vi "NXTLineLeader-DC.vi"(3 "Select your \nInput Port":T2 items=["Port 1", "Port 2", "Port 3", "Port 4"], 5 "NXT":T1={"error"={"status"=FALSE, "code"=0, "source"=""}, "address"="", "NXT #"=-1, "Show Error"=TRUE}) -> (17 "Boolean array":bool[](array[boolean]), 19 "NXT dup":T1={"error"={"status"=FALSE, "code"=0, "source"=""}, "address"="", "NXT #"=-1, "Show Error"=TRUE}, 20 "Sensor 1 Reading":u8, 21 "Sensor 2 Reading":u8, 22 "Sensor 3 Reading":u8, 23 "Sensor 4 Reading":u8, 24 "Sensor 5 Reading":u8, 25 "Sensor 6 Reading":u8, 26 "Sensor 7 Reading":u8, 27 "Sensor 8 Reading":u8)   [LabVIEW 2009]
uses:
  <vilib>/NXT/Block Support/NXT_InputPort.ctl
  <vilib>/NXT/Subs/LVHSConnector.ctl
  <vilib>/NXT/Block Support/HWPage.SensorType.ctl
  <vilib>/NXT/Block Support/HWPage.SensorMode.ctl
panel:
  # "mindsensors.com\nCopyright (c) 2009 by mindsensors.com\nEmail: info (<at>) mindsensors (<dot>) com\n\nThis program is free software. You can redistribute it and/or modify\nit under the terms of the GNU General Public License as published by\nthe Free Software Foundation; version 3 of the License.\nRead the license at: http://www.gnu.org/licenses/gpl.txt"
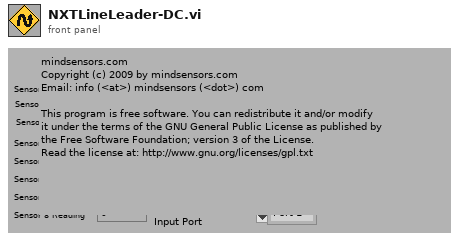
[diagram p1: front panel]
types:
  T1 = typedef "LVHSConnector.ctl" = cluster{"error":errorcluster, "address":string, "NXT #":i32, "Show Error":bool}
  T2 = typedef "NXT_InputPort.ctl" = u8
  T3 = typedef "HWPage.SensorMode.ctl" = u8
  T4 = typedef "HWPage.SensorType.ctl" = u8
  T5 = typedef "nxt.ctl" = cluster{"nxtHandle":u32, "fileHandle":u32, "fileIterHandle":u32, "moduleHandle":u32, "modIterHandle":u32, "nxtIterHandle":u32}
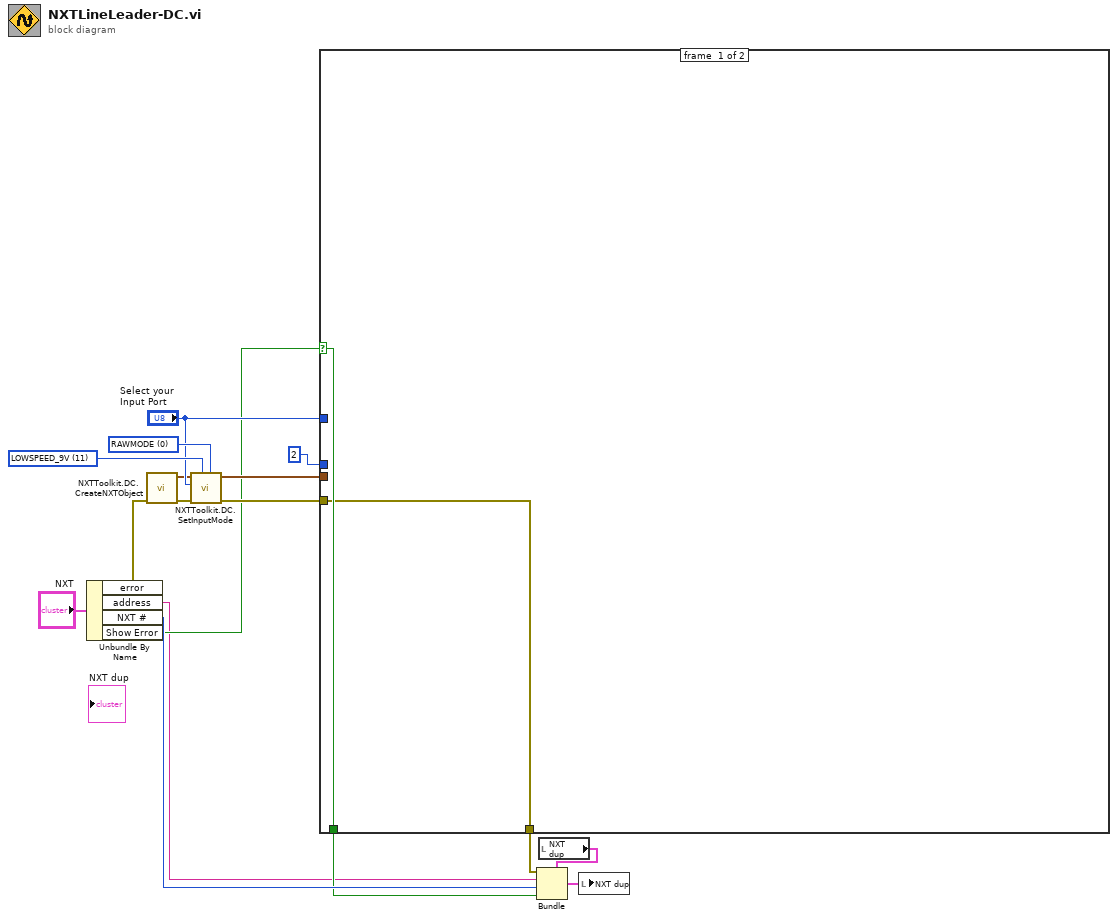
[diagram p0: block diagram]
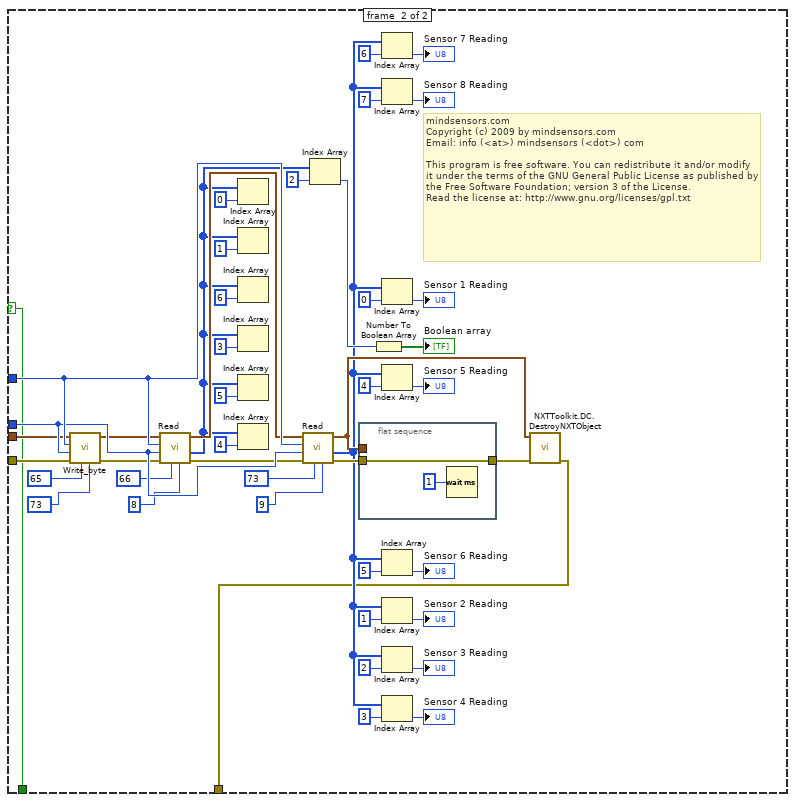
[diagram p2: hidden frame]
diagram:
  w15 = T3 0 items=["RAWMODE"=0, "BOOLEANMODE"=32, "TRANSITIONCNTMODE"=64, "PERIODCOUNTERMODE"=96, "PCTFULLSCALEMODE"=128, "CELSIUSMODE"=160, "FAHRENHEITMODE"=192, "ANGLESTEPMODE"=224] ("Sensor Mode (RAWMODE)")
  w16 = T4 11 items=["NO_SENSOR", "SWITCH", "TEMPERATURE", "REFLECTION", "ANGLE", "LIGHT_ACTIVE", "LIGHT_INACTIVE", "SOUND_DB", "SOUND_DBA", "CUSTOM", "LOWSPEED", "LOWSPEED_9V", "HIGHSPEED"] ("Sensor Type (NO_SENSOR)")
  n1 = Unbundle By Name("NXT") -> ("error"=w3:errorcluster, "address"=w4:string, "NXT #"=w7:i32, "Show Error"=w5:bool)
  n2 = call <vilib>:"NXTToolkit.DC.CreateNXTObject.vi"("error in (no error)"=w3) -> ("error out"=w17:errorcluster, "NXTObject"=w11:T5)  [unwired: 8 in, 1 out]
  n3 = call <vilib>:"NXTToolkit.DC.SetInputMode.vi"("Sensor Mode (RAWMODE)"=w15, "Sensor Type (NO_SENSOR)"=w16, "error in (no error)"=w17, "Input Port (Port 1)"="Select your \nInput Port", "NXTObject"=w11) -> ("error out"=w12:errorcluster, "NXTObject dup"=w13:T5)  [unwired: 4 in, 1 out]
  n4 = case shown="True" w5 {
    selector: w5 -> [w19 w21]
    tunnel: "Select your \nInput Port" -> [_ w63]
    tunnel: 2 -> [_ w62]
    tunnel: w13 -> [_ w59]
    tunnel: w12 -> [w18 w58]
    tunnel: [w19 w21] -> w6
    tunnel: [w18 w20] -> w2
    frame #0 {
    }
    frame #1 {
      # "mindsensors.com\nCopyright (c) 2009 by mindsensors.com\nEmail: info (<at>) mindsensors (<dot>) com\n\nThis program is free software. You can redistribute it and/or modify\nit under the terms of the GNU General Public License as published by\nthe Free Software Foundation; version 3 of the License.\nRead the license at: http://www.gnu.org/licenses/gpl.txt"
      n5 = call "Write_byte.vi"("Data byte"=73, "Reg Address"=u8 65, "error in (no error)"=w58, "Device Address"=w62, "Input Port in"=w63, "NXTObject"=w59) -> ("error out"=w60:errorcluster, "NXTObject dup"=w61:T5)  [unwired: 1 in, 3 out]
      n6 = call "Read.vi"("bytes to read"=u8 8, "Reg Address"=u8 66, "error in (no error)"=w60, "Device Address"=w62, "Input Port in"=w63, "NXTObject"=w61) -> ("error out"=w26:errorcluster, "data Buffer"=w24:u8[], "NXTObject dup"=w27:T5)  [unwired: 3 out]
      n7 = Index Array(array=w24, index=0) -> ()  [unwired: 1 out]
      n8 = Index Array(array=w24, index=1) -> ()  [unwired: 1 out]
      n9 = Index Array(array=w24, index=6) -> ()  [unwired: 1 out]
      n10 = Index Array(array=w24, index=3) -> ()  [unwired: 1 out]
      n11 = Index Array(array=w24, index=5) -> ()  [unwired: 1 out]
      n12 = Index Array(array=w24, index=4) -> ()  [unwired: 1 out]
      n13 = call "Read.vi"("bytes to read"=u8 9, "Reg Address"=u8 73, "error in (no error)"=w26, "Device Address"=w62, "Input Port in"=w63, "NXTObject"=w27) -> ("error out"=w52:errorcluster, "data Buffer"=w23:u8[], "NXTObject dup"=w57:T5)  [unwired: 3 out]
      n14 = Index Array(array=w24, index=2) -> (element=w36:u8)
      n15 = flat-sequence {
        tunnel: [w66] -> w22
        tunnel: w52 -> [w66]
        tunnel: w57 -> [_]
        frame #0 {
          n16 = Wait (ms)(milliseconds to wait=u32 1) -> ()  [unwired: 1 out]
        }
      }
      n17 = Number To Boolean Array(number=w36) -> (Boolean array=→"Boolean array":bool[])
      n18 = Index Array(array=w23, index=6) -> (element=→"Sensor 7 Reading":u8)
      n19 = Index Array(array=w23, index=7) -> (element=→"Sensor 8 Reading":u8)
      n20 = Index Array(array=w23, index=0) -> (element=→"Sensor 1 Reading":u8)
      n21 = Index Array(array=w23, index=4) -> (element=→"Sensor 5 Reading":u8)
      n22 = Index Array(array=w23, index=5) -> (element=→"Sensor 6 Reading":u8)
      n23 = Index Array(array=w23, index=1) -> (element=→"Sensor 2 Reading":u8)
      n24 = Index Array(array=w23, index=2) -> (element=→"Sensor 3 Reading":u8)
      n25 = Index Array(array=w23, index=3) -> (element=→"Sensor 4 Reading":u8)
      n26 = call <vilib>:"NXTToolkit.DC.DestroyNXTObject.vi"("error in (no error)"=w22, "NXTObject"=w57) -> ("error out"=w20:errorcluster)  [unwired: 9 in]
    }
  }
  n27 = local read "NXT dup"() -> (w8:T1)
  n28 = Bundle(cluster=w8, "error"=w2, "address"=w4, "NXT #"=w7, "Show Error"=w6) -> (w9:T1)
  n29 = local write "NXT dup"(w9) -> ()
